vi "Cursor_Control.vi"(5 "Channel 1 EN":bool, 7 "Channel 0 EN":bool, 9 "Cursor1 ON":bool, 10 "Curso0 ON":bool, 11 "WaveformGraph in":refnum<vi>) -> (0 "Cursor0_Scale1_disp":string, 1 "Delta Ch0":string, 2 "Cursor1_Scale0_disp":string, 3 "Cursor0_Scale0_disp":string, 4 "Cursor1_Scale1_disp":string, 6 "Delta Ch1":string)   [LabVIEW 2019]
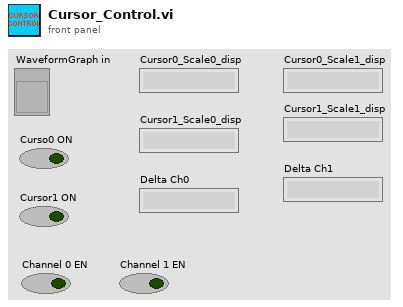
[diagram p1: front panel]
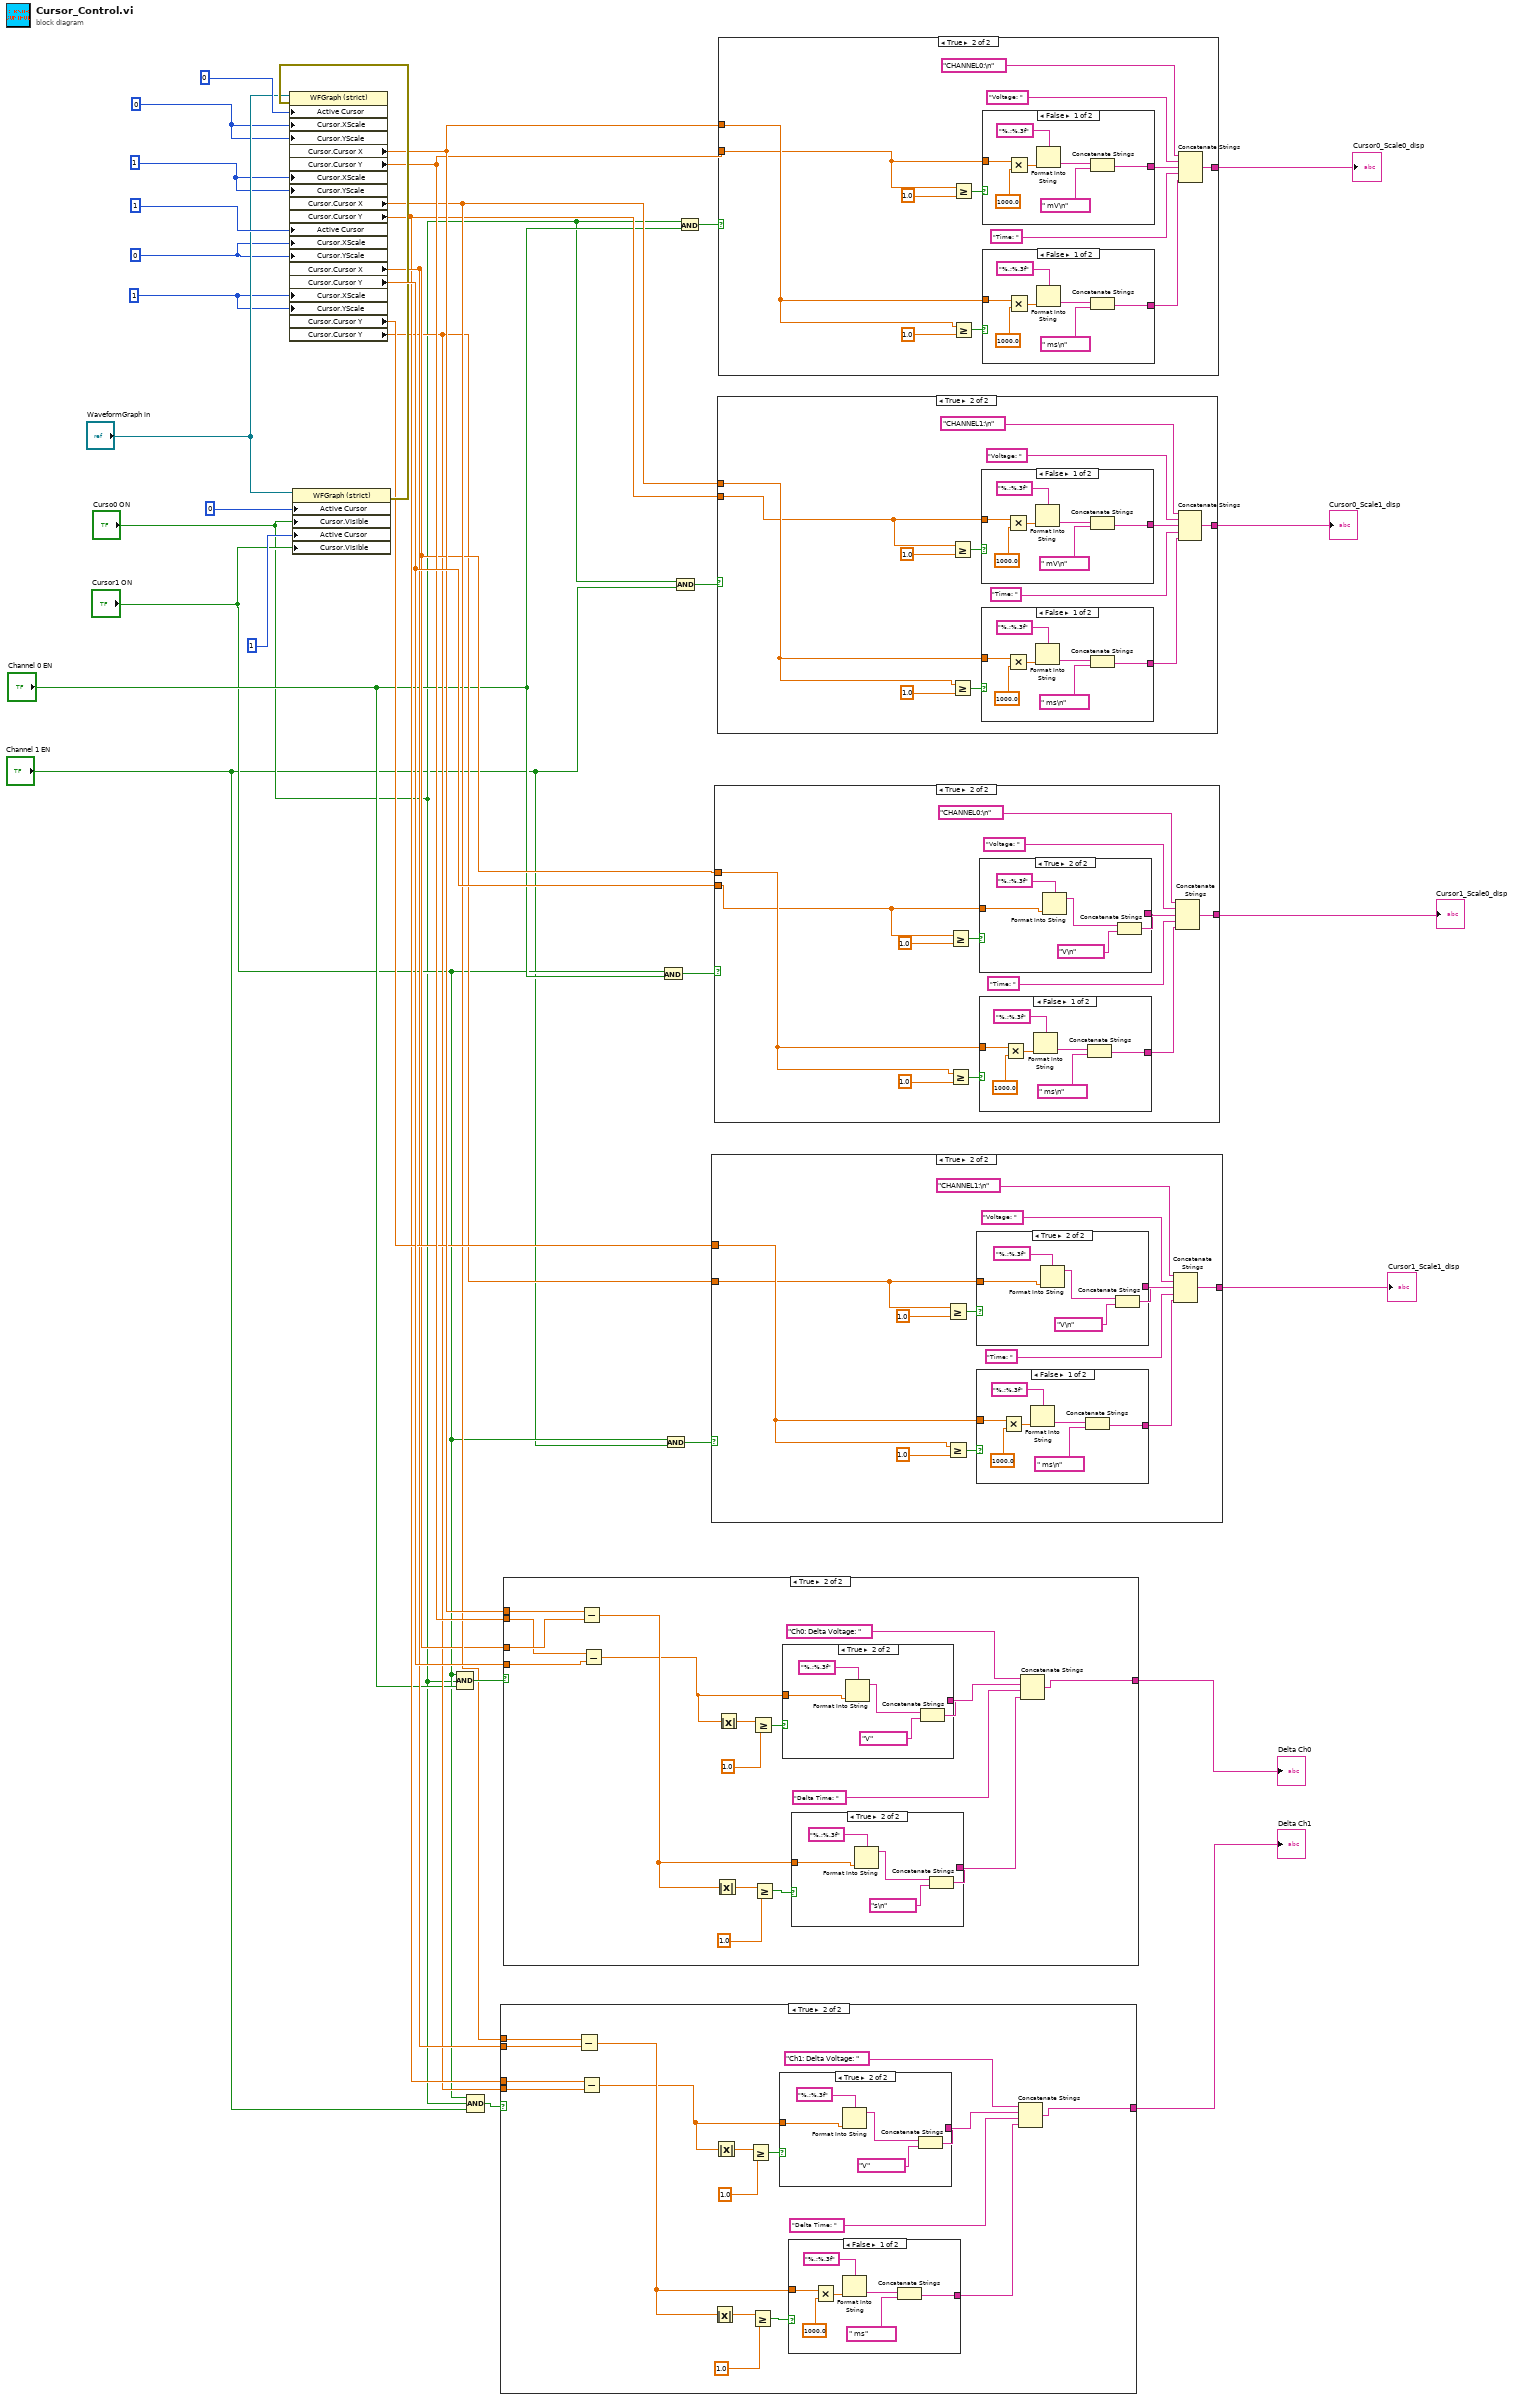
[diagram p0: block diagram]
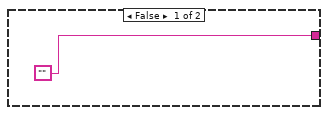
[diagram p2: hidden frame]
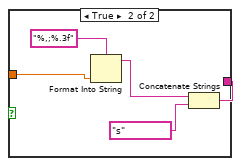
[diagram p3: hidden frame]
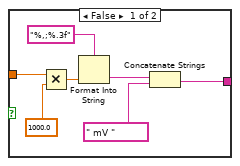
[diagram p4: hidden frame]
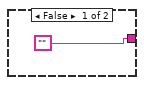
[diagram p5: hidden frame]
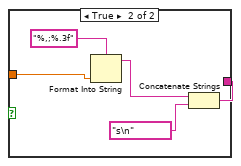
[diagram p6: hidden frame]
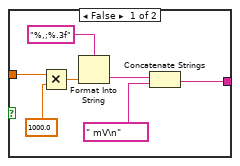
[diagram p7: hidden frame]
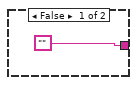
[diagram p8: hidden frame]
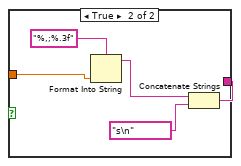
[diagram p9: hidden frame]
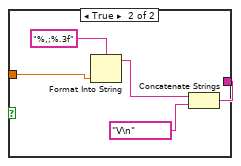
[diagram p10: hidden frame]
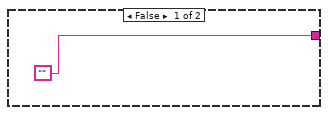
[diagram p11: hidden frame]
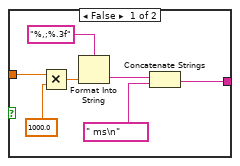
[diagram p12: hidden frame]
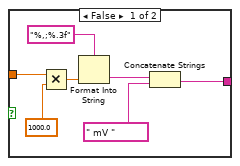
[diagram p13: hidden frame]
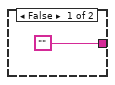
[diagram p14: hidden frame]
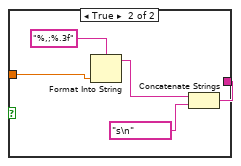
[diagram p15: hidden frame]
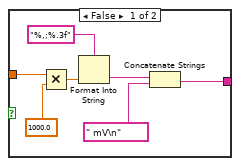
[diagram p16: hidden frame]
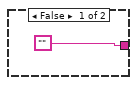
[diagram p17: hidden frame]
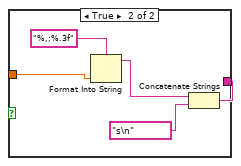
[diagram p18: hidden frame]
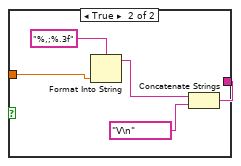
[diagram p19: hidden frame]
diagram:
  w17 = u32 0 ("Cursor.X Scale")
  w18 = u32 1 ("Cursor.X Scale")
  w19 = 1 ("Cursor.Cursor Plot")
  w20 = 0 ("Cursor.Cursor Plot")
  n1 = property on="Property Node" class="WFGraph (strict)"(reference="WaveformGraph in", "Active Cursor"=u32 0, "Cursor.Visible"="Curso0 ON", "Active Cursor"=u32 1, "Cursor.Visible"="Cursor1 ON") -> (error out=w28:errorcluster)  [unwired: 1 in, 1 out]
  n2 = property on="Property Node" class="WFGraph (strict)"(reference="WaveformGraph in", error in=w28, "Active Cursor"=u32 0, "Cursor.XScale"=w20, "Cursor.YScale"=w20, "Cursor.XScale"=w19, "Cursor.YScale"=w19, "Active Cursor"=u32 1, "Cursor.XScale"=w17, "Cursor.YScale"=w17, "Cursor.XScale"=w18, "Cursor.YScale"=w18) -> ("Cursor.Cursor X"=w23:dbl, "Cursor.Cursor Y"=w22:dbl, "Cursor.Cursor X"=w9:dbl, "Cursor.Cursor Y"=w7:dbl, "Cursor.Cursor X"=w8:dbl, "Cursor.Cursor Y"=w34:dbl, "Cursor.Cursor Y"=w16:dbl, "Cursor.Cursor Y"=w6:dbl)  [unwired: 2 out]
  n3 = Compound Arithmetic op=AND("Cursor1 ON", "Curso0 ON", "Channel 0 EN") -> (w33:bool)
  n4 = Compound Arithmetic op=AND("Cursor1 ON", "Curso0 ON", "Channel 1 EN") -> (w1:bool)
  n5 = case shown="True" w1 {
    tunnel: ["" w44] -> w10
    tunnel: w9 -> [_ w39]
    tunnel: w8 -> [_ w38]
    tunnel: w7 -> [_ w37]
    tunnel: w6 -> [_ w36]
    frame False {
    }
    frame True {
      n6 = Subtract(x=w39, y=w38) -> (x-y=w42:dbl)
      n7 = Subtract(x=w37, y=w36) -> (x-y=w40:dbl)
      n8 = Absolute Value(x=w42) -> (abs(x)=w43:dbl)
      n9 = Absolute Value(x=w40) -> (abs(x)=w41:dbl)
      n10 = Greater Or Equal?(x=w41, y=1.0) -> (x >= y?=w52:bool)
      n11 = Greater Or Equal?(x=w43, y=1.0) -> (x >= y?=w48:bool)
      n12 = case shown="True" w52 {
        tunnel: [w66 w73] -> w49
        tunnel: w40 -> [w65 w72]
        frame False {
          n13 = Multiply(x=w65, y=1000.0) -> (x*y=w67:dbl)
          n14 = Format Into String(format string="%,;%.3f", w67) -> (resulting string=w70:string)  [unwired: 2 in, 1 out]
          n15 = Concatenate Strings(w70, " mV ") -> (w66:string)
        }
        frame True {
          n16 = Format Into String(format string="%,;%.3f", w72) -> (resulting string=w76:string)  [unwired: 2 in, 1 out]
          n17 = Concatenate Strings(w76, "V") -> (w73:string)
        }
      }
      n18 = case shown="False" w48 {
        tunnel: [w54 w61] -> w46
        tunnel: w42 -> [w53 w60]
        frame False {
          n19 = Multiply(x=w53, y=1000.0) -> (x*y=w55:dbl)
          n20 = Format Into String(format string="%,;%.3f", w55) -> (resulting string=w58:string)  [unwired: 2 in, 1 out]
          n21 = Concatenate Strings(w58, " ms") -> (w54:string)
        }
        frame True {
          n22 = Format Into String(format string="%,;%.3f", w60) -> (resulting string=w64:string)  [unwired: 2 in, 1 out]
          n23 = Concatenate Strings(w64, "s") -> (w61:string)
        }
      }
      n24 = Concatenate Strings("Ch1: Delta Voltage: ", w49, "Delta Time: ", w46) -> (w44:string)
    }
  }
  "Delta Ch1" <- w10
  n25 = case shown="True" w33 {
    tunnel: w23 -> [_ w94]
    tunnel: w22 -> [_ w92]
    tunnel: w8 -> [_ w93]
    tunnel: w34 -> [_ w91]
    tunnel: ["" w82] -> w24
    frame False {
    }
    frame True {
      n26 = Subtract(x=w94, y=w93) -> (x-y=w80:dbl)
      n27 = Subtract(x=w92, y=w91) -> (x-y=w78:dbl)
      n28 = Absolute Value(x=w80) -> (abs(x)=w81:dbl)
      n29 = Absolute Value(x=w78) -> (abs(x)=w79:dbl)
      n30 = Greater Or Equal?(x=w79, y=1.0) -> (x >= y?=w90:bool)
      n31 = Greater Or Equal?(x=w81, y=1.0) -> (x >= y?=w86:bool)
      n32 = case shown="True" w90 {
        tunnel: [w108 w115] -> w87
        tunnel: w78 -> [w107 w114]
        frame False {
          n33 = Multiply(x=w107, y=1000.0) -> (x*y=w109:dbl)
          n34 = Format Into String(format string="%,;%.3f", w109) -> (resulting string=w112:string)  [unwired: 2 in, 1 out]
          n35 = Concatenate Strings(w112, " mV ") -> (w108:string)
        }
        frame True {
          n36 = Format Into String(format string="%,;%.3f", w114) -> (resulting string=w118:string)  [unwired: 2 in, 1 out]
          n37 = Concatenate Strings(w118, "V") -> (w115:string)
        }
      }
      n38 = case shown="True" w86 {
        tunnel: [w96 w103] -> w84
        tunnel: w80 -> [w95 w102]
        frame False {
          n39 = Multiply(x=w95, y=1000.0) -> (x*y=w97:dbl)
          n40 = Format Into String(format string="%,;%.3f", w97) -> (resulting string=w100:string)  [unwired: 2 in, 1 out]
          n41 = Concatenate Strings(w100, " ms\n") -> (w96:string)
        }
        frame True {
          n42 = Format Into String(format string="%,;%.3f", w102) -> (resulting string=w106:string)  [unwired: 2 in, 1 out]
          n43 = Concatenate Strings(w106, "s\n") -> (w103:string)
        }
      }
      n44 = Concatenate Strings("Ch0: Delta Voltage: ", w87, "Delta Time: ", w84) -> (w82:string)
    }
  }
  "Delta Ch0" <- w24
  n45 = And(x="Cursor1 ON", y="Channel 0 EN") -> (x .and. y?=w12:bool)
  n46 = And(x="Cursor1 ON", y="Channel 1 EN") -> (x .and. y?=w11:bool)
  n47 = And(x="Curso0 ON", y="Channel 1 EN") -> (x .and. y?=w14:bool)
  n48 = And(x="Curso0 ON", y="Channel 0 EN") -> (x .and. y?=w13:bool)
  n49 = case shown="True" w11 {
    tunnel: w16 -> [_ w122]
    tunnel: w6 -> [_ w121]
    tunnel: ["" w120] -> w15
    frame False {
    }
    frame True {
      n50 = Greater Or Equal?(x=w121, y=1.0) -> (x >= y?=w126:bool)
      n51 = Greater Or Equal?(x=w122, y=1.0) -> (x >= y?=w124:bool)
      n52 = case shown="True" w126 {
        tunnel: [w145 w152] -> w125
        tunnel: w121 -> [w144 w151]
        frame False {
          n53 = Multiply(x=w144, y=1000.0) -> (x*y=w146:dbl)
          n54 = Format Into String(format string="%,;%.3f", w146) -> (resulting string=w149:string)  [unwired: 2 in, 1 out]
          n55 = Concatenate Strings(w149, " mV\n") -> (w145:string)
        }
        frame True {
          n56 = Format Into String(format string="%,;%.3f", w151) -> (resulting string=w155:string)  [unwired: 2 in, 1 out]
          n57 = Concatenate Strings(w155, "V\n") -> (w152:string)
        }
      }
      n58 = case shown="False" w124 {
        tunnel: [w133 w140] -> w123
        tunnel: w122 -> [w132 w139]
        frame False {
          n59 = Multiply(x=w132, y=1000.0) -> (x*y=w134:dbl)
          n60 = Format Into String(format string="%,;%.3f", w134) -> (resulting string=w137:string)  [unwired: 2 in, 1 out]
          n61 = Concatenate Strings(w137, " ms\n") -> (w133:string)
        }
        frame True {
          n62 = Format Into String(format string="%,;%.3f", w139) -> (resulting string=w143:string)  [unwired: 2 in, 1 out]
          n63 = Concatenate Strings(w143, "s\n") -> (w140:string)
        }
      }
      n64 = Concatenate Strings("CHANNEL1:\n", "Voltage: ", w125, "Time: ", w123) -> (w120:string)
    }
  }
  "Cursor1_Scale1_disp" <- w15
  n65 = case shown="True" w12 {
    tunnel: w8 -> [_ w158]
    tunnel: w34 -> [_ w157]
    tunnel: ["" w159] -> w32
    frame False {
    }
    frame True {
      n66 = Greater Or Equal?(x=w157, y=1.0) -> (x >= y?=w165:bool)
      n67 = Greater Or Equal?(x=w158, y=1.0) -> (x >= y?=w167:bool)
      n68 = case shown="True" w165 {
        tunnel: [w182 w189] -> w166
        tunnel: w157 -> [w181 w188]
        frame False {
          n69 = Multiply(x=w181, y=1000.0) -> (x*y=w183:dbl)
          n70 = Format Into String(format string="%,;%.3f", w183) -> (resulting string=w186:string)  [unwired: 2 in, 1 out]
          n71 = Concatenate Strings(w186, " mV\n") -> (w182:string)
        }
        frame True {
          n72 = Format Into String(format string="%,;%.3f", w188) -> (resulting string=w192:string)  [unwired: 2 in, 1 out]
          n73 = Concatenate Strings(w192, "V\n") -> (w189:string)
        }
      }
      n74 = case shown="False" w167 {
        tunnel: [w170 w177] -> w168
        tunnel: w158 -> [w169 w176]
        frame False {
          n75 = Multiply(x=w169, y=1000.0) -> (x*y=w171:dbl)
          n76 = Format Into String(format string="%,;%.3f", w171) -> (resulting string=w174:string)  [unwired: 2 in, 1 out]
          n77 = Concatenate Strings(w174, " ms\n") -> (w170:string)
        }
        frame True {
          n78 = Format Into String(format string="%,;%.3f", w176) -> (resulting string=w180:string)  [unwired: 2 in, 1 out]
          n79 = Concatenate Strings(w180, "s\n") -> (w177:string)
        }
      }
      n80 = Concatenate Strings("CHANNEL0:\n", "Voltage: ", w166, "Time: ", w168) -> (w159:string)
    }
  }
  "Cursor1_Scale0_disp" <- w32
  n81 = case shown="True" w14 {
    tunnel: w9 -> [_ w195]
    tunnel: w7 -> [_ w194]
    tunnel: ["" w196] -> w21
    frame False {
    }
    frame True {
      n82 = Greater Or Equal?(x=w194, y=1.0) -> (x >= y?=w202:bool)
      n83 = Greater Or Equal?(x=w195, y=1.0) -> (x >= y?=w204:bool)
      n84 = case shown="False" w202 {
        tunnel: [w219 w226] -> w203
        tunnel: w194 -> [w218 w225]
        frame False {
          n85 = Multiply(x=w218, y=1000.0) -> (x*y=w220:dbl)
          n86 = Format Into String(format string="%,;%.3f", w220) -> (resulting string=w223:string)  [unwired: 2 in, 1 out]
          n87 = Concatenate Strings(w223, " mV\n") -> (w219:string)
        }
        frame True {
          n88 = Format Into String(format string="%,;%.3f", w225) -> (resulting string=w229:string)  [unwired: 2 in, 1 out]
          n89 = Concatenate Strings(w229, "V\n") -> (w226:string)
        }
      }
      n90 = case shown="False" w204 {
        tunnel: [w207 w214] -> w205
        tunnel: w195 -> [w206 w213]
        frame False {
          n91 = Multiply(x=w206, y=1000.0) -> (x*y=w208:dbl)
          n92 = Format Into String(format string="%,;%.3f", w208) -> (resulting string=w211:string)  [unwired: 2 in, 1 out]
          n93 = Concatenate Strings(w211, " ms\n") -> (w207:string)
        }
        frame True {
          n94 = Format Into String(format string="%,;%.3f", w213) -> (resulting string=w217:string)  [unwired: 2 in, 1 out]
          n95 = Concatenate Strings(w217, "s\n") -> (w214:string)
        }
      }
      n96 = Concatenate Strings("CHANNEL1:\n", "Voltage: ", w203, "Time: ", w205) -> (w196:string)
    }
  }
  "Cursor0_Scale1_disp" <- w21
  n97 = case shown="True" w13 {
    tunnel: w23 -> [_ w232]
    tunnel: w22 -> [_ w231]
    tunnel: ["" w233] -> w31
    frame False {
    }
    frame True {
      n98 = Greater Or Equal?(x=w231, y=1.0) -> (x >= y?=w239:bool)
      n99 = Greater Or Equal?(x=w232, y=1.0) -> (x >= y?=w241:bool)
      n100 = case shown="False" w239 {
        tunnel: [w256 w263] -> w240
        tunnel: w231 -> [w255 w262]
        frame False {
          n101 = Multiply(x=w255, y=1000.0) -> (x*y=w257:dbl)
          n102 = Format Into String(format string="%,;%.3f", w257) -> (resulting string=w260:string)  [unwired: 2 in, 1 out]
          n103 = Concatenate Strings(w260, " mV\n") -> (w256:string)
        }
        frame True {
          n104 = Format Into String(format string="%,;%.3f", w262) -> (resulting string=w266:string)  [unwired: 2 in, 1 out]
          n105 = Concatenate Strings(w266, "V\n") -> (w263:string)
        }
      }
      n106 = case shown="False" w241 {
        tunnel: [w244 w251] -> w242
        tunnel: w232 -> [w243 w250]
        frame False {
          n107 = Multiply(x=w243, y=1000.0) -> (x*y=w245:dbl)
          n108 = Format Into String(format string="%,;%.3f", w245) -> (resulting string=w248:string)  [unwired: 2 in, 1 out]
          n109 = Concatenate Strings(w248, " ms\n") -> (w244:string)
        }
        frame True {
          n110 = Format Into String(format string="%,;%.3f", w250) -> (resulting string=w254:string)  [unwired: 2 in, 1 out]
          n111 = Concatenate Strings(w254, "s\n") -> (w251:string)
        }
      }
      n112 = Concatenate Strings("CHANNEL0:\n", "Voltage: ", w240, "Time: ", w242) -> (w233:string)
    }
  }
  "Cursor0_Scale0_disp" <- w31
